vi "TCP testing.vi"() -> ()   [LabVIEW 2019]
panel:
  out "data out 2":string
  out "data out":string
  out "error out":errorcluster
  in  "error in (no error)":errorcluster
  in  "address":string="192.168.3.1"
  in  "remote port or service name":u16=1025
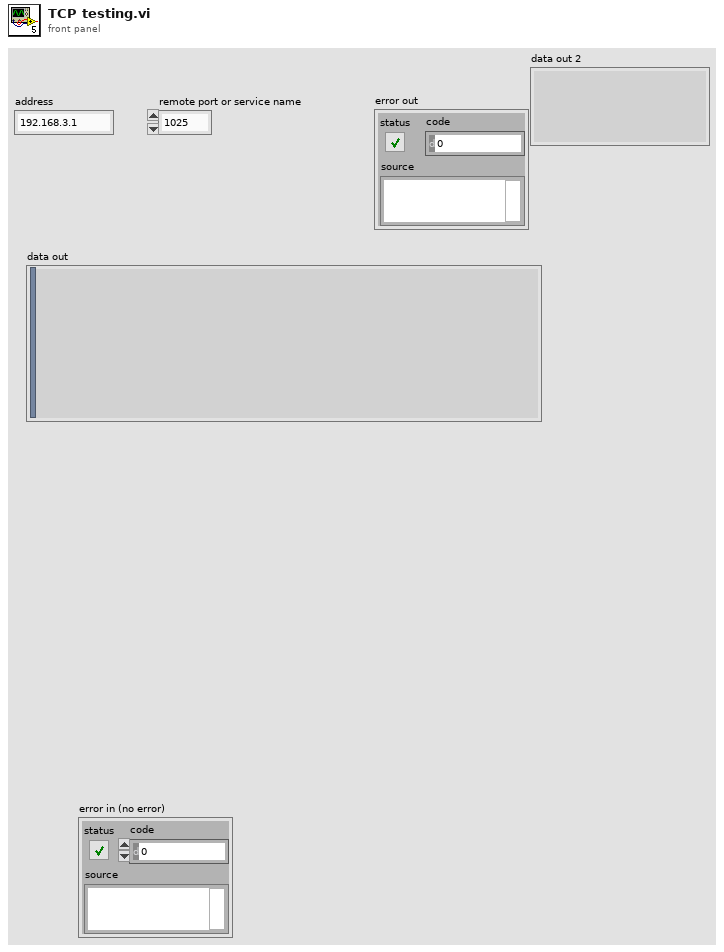
[diagram p1: front panel]
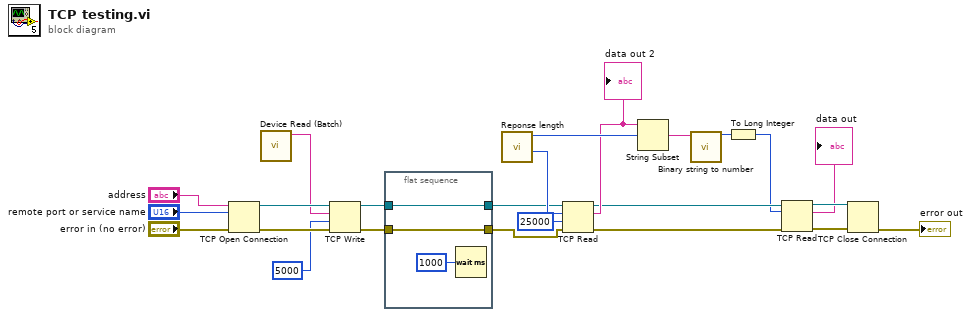
[diagram p0: block diagram]
diagram:
  n1 = TCP Open Connection(address="address", remote port or service name="remote port or service name", error in (no error)="error in (no error)") -> (connection ID=w21:refnum<k5>, error out=w20:errorcluster)  [unwired: 2 in]
  n2 = call "Device Read (Batch).vi"() -> ("Device Read (Batch) string"=w19:string)  [unwired: 11 in]
  n3 = TCP Write(connection ID=w21, data in=w19, error in (no error)=w20, 9:5000 ("timeout ms (25000)")) -> (connection ID out=w4:refnum<k5>, error out=w3:errorcluster)  [unwired: 1 out]
  n4 = flat-sequence {
    tunnel: w4 -> [w27]
    tunnel: w3 -> [w26]
    tunnel: [w27] -> w2
    tunnel: [w26] -> w1
    frame #0 {
      n5 = Wait (ms)(milliseconds to wait=u32 1000) -> ()  [unwired: 1 out]
    }
  }
  n6 = call "Reponse length.vi"() -> ("headers length include length"=w18:i32, "headers length"=w17:i32)  [unwired: 10 in]
  n7 = TCP Read(connection ID=w2, bytes to read=w18, error in (no error)=w1, 9:25000 ("timeout ms (25000)")) -> (connection ID out=w15:refnum<k5>, data out=w16:string, error out=w14:errorcluster)  [unwired: 1 in]
  "data out 2" <- w16
  n8 = String Subset(string=w16, offset (0)=w17) -> (substring=w13:string)  [unwired: 1 in]
  n9 = call "Binary string to number.vi"("Binaty string"=w13) -> ("Numeric"=w12:u32)  [unwired: 10 in]
  n10 = To Long Integer(number=w12) -> (32bit integer=w11:i32)
  n11 = TCP Read(connection ID=w15, bytes to read=w11, error in (no error)=w14) -> (connection ID out=w8:refnum<k5>, data out=→"data out":string, error out=w7:errorcluster)  [unwired: 2 in]
  n12 = TCP Close Connection(connection ID=w8, error in (no error)=w7) -> (error out=→"error out":errorcluster)  [unwired: 1 in, 1 out]
